vi "SCCAPI Open Project.vi"(8 "error in (no error)":errorcluster, 11 "configuration data":string) -> (0 "error out":errorcluster, 2 "status message":string, 3 "source control reference out":T1)   [LabVIEW 2017, in "NI_SCC.lvlib"]
uses:
  <vilib>/SourceControl/sccapi/NI_SCC.lvlib
  <vilib>/SourceControl/sccapi/SCCAPI Refnum.ctl
  <vilib>/SourceControl/sccapi/SCCAPI SCC Operations.ctl
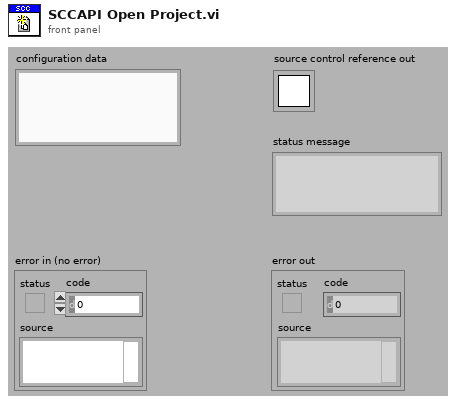
[diagram p1: front panel]
types:
  T1 = typedef "NI_SCC.lvlib/SCCAPI Refnum.ctl" = refnum<k1>
  T2 = typedef "NI_SCC.lvlib/SCCAPI SCC Operations.ctl" = enum16{"Add", "Check In", "Check Out", "Close Project", "Compare Files", "Compare VIs", "Configure Project", "File History", "File Properties", "File Status", "Find All Providers", "Get Advanced Command Options", "Get File Copy", "Get Latest Version", "Get Project Name", "Get StaticVI Path", "Initialize", "Not A Source Control Reference", "Open Project", "Provider Supports Functionality", "Remove", "Run Provider", "Undo Check Out", "Uninitialize", "Is File In Local Path"}
  T3 = typedef "SCCAPI Refnum.ctl" = refnum<k1>
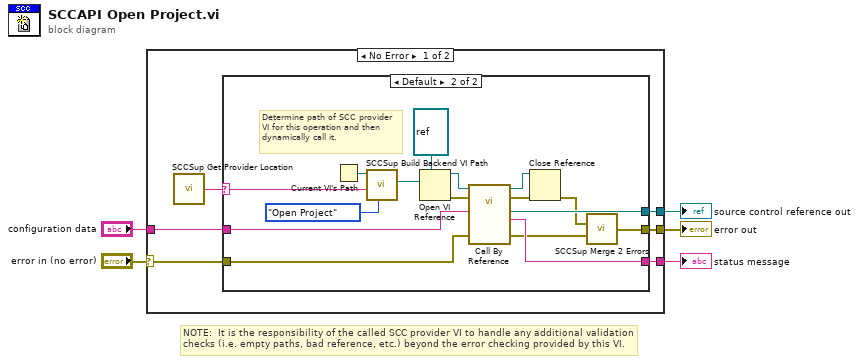
[diagram p0: block diagram]
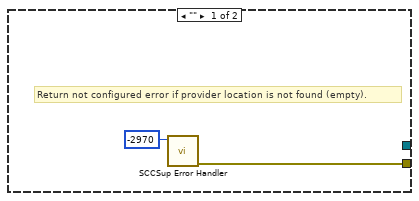
[diagram p2: hidden frame]
diagram:
  # "NOTE:  It is the responsibility of the called SCC provider VI to handle any additional validation checks (i.e. empty paths, bad reference, etc.) beyond the error checking provided by this VI."
  n1 = case shown="No Error" "error in (no error)" {
    selector: "error in (no error)" -> [w7 w30]
    tunnel: [w11 w30] -> w4
    tunnel: [w10 _] -> w3
    tunnel: [w9 _] -> w2
    tunnel: "configuration data" -> [w6 _]
    frame No Error {
      n2 = call <vilib>:"SCCSup Get Provider Location.vi"() -> ("provider location"=w8:string)  [unwired: 6 in]
      n3 = case shown="Default" w8 {
        selector: w8 -> [_ w16]
        tunnel: [w12 w27] -> w11
        tunnel: [_ w21] -> w10
        tunnel: [_ w20] -> w9
        tunnel: w7 -> [_ w15]
        tunnel: w6 -> [_ w14]
        frame "" {
          # "Return not configured error if provider location is not found (empty)."
          n4 = call <vilib>:"SCCSup Error Handler.vi"("scc error code"=-2970 ("code")) -> ("error out"=w12:errorcluster)  [unwired: 10 in]
        }
        frame Default {
          # "Determine path of SCC provider VI for this operation and then dynamically call it."
          n5 = Current VI's Path() -> (path=w28:path)
          n6 = call <vilib>:"SCCSup Build Backend VI Path.vi"("scc operation"=SCCAPI_SCC_Operations."Open Project", "provider location"=w16, "caller path"=w28) -> ("scc backend VI path"=w29:path)  [unwired: 8 in]
          n7 = Open VI Reference(type specifier VI Refnum (for type only)=refnum<vi> refnum, vi path=w29) -> (vi reference=w25:refnum<vi>, error out=w24:errorcluster)  [unwired: 4 in]
          n8 = call-by-ref "?"(reference=w25, error in=w24, "error in (no error)"=w15, "configuration data"=w14) -> (reference out=w23:refnum<vi>, error out=w22:errorcluster, 0:"error out"=w18:errorcluster, "status message"=w21:string, "source control reference out"=w20:T3)  [unwired: 7 in]
          n9 = Close Reference(reference=w23, error in (no error)=w22) -> (error out=w19:errorcluster)
          n10 = call <vilib>:"SCCSup Merge 2 Errors.vi"("Error IO 1"=w19, "Error IO 2"=w18) -> ("Error IO out"=w27:errorcluster)  [unwired: 13 in]
        }
      }
    }
    frame Error {
    }
  }
  "error out" <- w4
  "status message" <- w3
  "source control reference out" <- w2
